vi "E2_Chart1.vi"() -> ()   [LabVIEW 2020]
panel:
  in  "stop":bool
  in  "Delay (ms)":dbl(slide) scale=0.0..100.0
  out "Waveform Chart":dbl(graph)
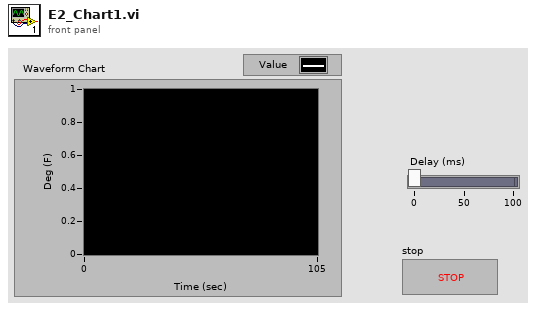
[diagram p1: front panel]
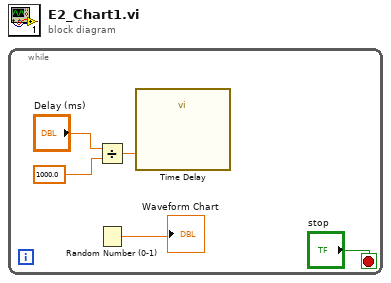
[diagram p0: block diagram]
diagram:
  n1 = while {
    stop <- "stop" stop-if-true
    n2 = Divide(x="Delay (ms)", y=1000.0) -> (x/y=w3:dbl)
    n3 = Random Number (0-1)() -> (number: 0 to 1=→"Waveform Chart":dbl)
    n4 = call "Time Delay"("Delay Time (s)"=w3) -> ()  [unwired: 10 in, 1 out]
  }
